vi "AutoChooseState.vi"(8 "error in (no error)":errorcluster, 9 "HotGoal?":bool, 10 "AutoMode":T2, 11 "AutoState":T1) -> (0 "error out":errorcluster, 3 "AutoState":T1)   [LabVIEW 2013]
uses:
  AutoStates.ctl
  AutoMode.ctl
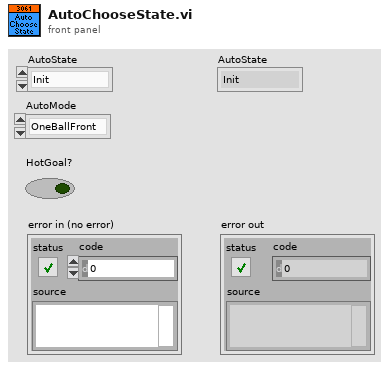
[diagram p1: front panel]
types:
  T1 = typedef "AutoStates.ctl" = enum16{"Init", "LowerArmCheckGoal", "DriveBack", "Collect", "StopCollect", "LiftArm", "RaiseServo", "Drive", "ShouldWait", "Wait", "ShootCollectorUp", "RaiseArm", "ShootCollectorDown", "Rotate1", "Rotate2", "Stop"}
  T2 = typedef "AutoMode.ctl" = enum16{"OneBallFront", "OneBallCollector", "TwoBallNormal", "TwoBallHot"}
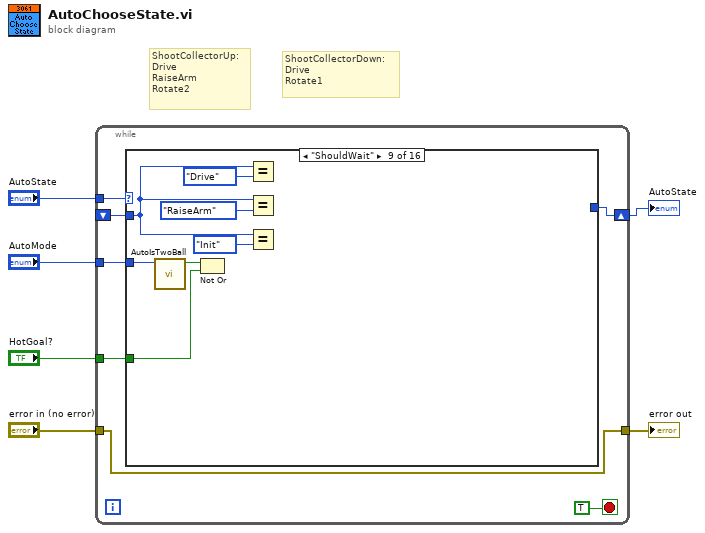
[diagram p0: block diagram]
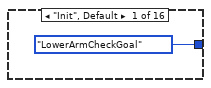
[diagram p2: hidden frame]
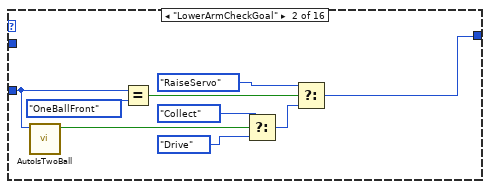
[diagram p3: hidden frame]
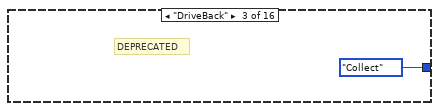
[diagram p4: hidden frame]
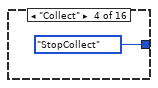
[diagram p5: hidden frame]
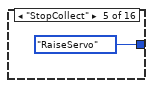
[diagram p6: hidden frame]
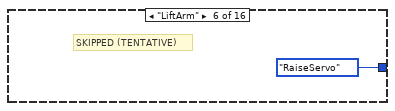
[diagram p7: hidden frame]
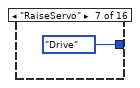
[diagram p8: hidden frame]
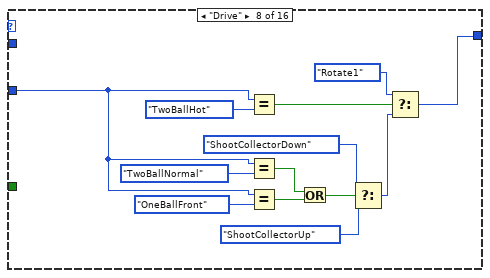
[diagram p9: hidden frame]
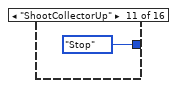
[diagram p11: hidden frame]
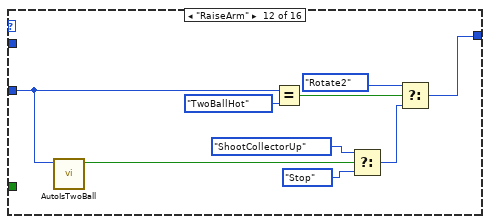
[diagram p12: hidden frame]
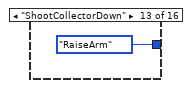
[diagram p13: hidden frame]
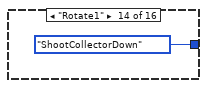
[diagram p14: hidden frame]
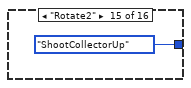
[diagram p15: hidden frame]
diagram:
  # "ShootCollectorDown:\nDrive\nRotate1"
  # "ShootCollectorUp:\nDrive\nRaiseArm\nRotate2"
  n1 = while {
    tunnel: "AutoMode" -> [w13]
    tunnel: "AutoState" -> [w12]
    tunnel: "HotGoal?" -> [w11]
    tunnel: "error in (no error)" -> [w8]
    tunnel: [w8] -> w1
    shift-right: [w10] -> w3
    shift-left: _ -> [w7]
    stop <- TRUE stop-if-true
    n2 = case shown="\"ShouldWait\"" w12 {
      selector: w12 -> [_ _ _ _ _ _ _ _ _ _ _ _ _ _ _ w62]
      tunnel: w13 -> [_ w17 _ _ _ _ _ w29 w48 _ _ w50 _ _ _ _]
      tunnel: w11 -> [_ _ _ _ _ _ _ _ w46 _ _ _ _ _ _ _]
      tunnel: [AutoStates."LowerArmCheckGoal" ("AutoState") w15 AutoStates."Collect" ("Enum") AutoStates."StopCollect" ("Enum") AutoStates."RaiseServo" ("Enum") AutoStates."RaiseServo" ("Enum") AutoStates."Drive" ("Enum") w31 _ _ AutoStates."Stop" ("f") w54 AutoStates."RaiseArm" ("Enum") AutoStates."ShootCollectorDown" ("Enum") AutoStates."ShootCollectorUp" ("Enum") w62] -> w10
      tunnel: w7 -> [_ _ _ _ _ _ _ _ w45 _ _ _ _ _ _ _]
      frame "Init", Default {
      }
      frame "LowerArmCheckGoal" {
        n3 = call "AutoIsTwoBall.vi"("AutoMode"=w17) -> ("IsTwoBall?"=w16:bool)  [unwired: 10 in]
        n4 = Equal?(x=w17, y=AutoMode."OneBallFront") -> (x = y?=w18:bool)
        n5 = Select(t=AutoStates."Collect" ("Enum"), s=w16, f=AutoStates."Drive" ("Enum")) -> (s? t:f=w20:T1)
        n6 = Select(t=AutoStates."RaiseServo" ("Enum"), s=w18, f=w20) -> (s? t:f=w15:T1)
      }
      frame "DriveBack" {
        # "DEPRECATED"
      }
      frame "Collect" {
      }
      frame "StopCollect" {
      }
      frame "LiftArm" {
        # "SKIPPED (TENTATIVE)"
      }
      frame "RaiseServo" {
      }
      frame "Drive" {
        n7 = Equal?(x=w29, y=AutoMode."TwoBallHot") -> (x = y?=w33:bool)
        n8 = Equal?(x=w29, y=AutoMode."TwoBallNormal") -> (x = y?=w40:bool)
        n9 = Equal?(x=w29, y=AutoMode."OneBallFront") -> (x = y?=w39:bool)
        n10 = Or(x=w40, y=w39) -> (x .or. y?=w35:bool)
        n11 = Select(t=AutoStates."ShootCollectorDown" ("Enum"), s=w35, f=AutoStates."ShootCollectorUp") -> (s? t:f=w34:T1)
        n12 = Select(t=AutoStates."Rotate1" ("Enum"), s=w33, f=w34) -> (s? t:f=w31:T1)
      }
      frame "ShouldWait" {
        n13 = call "AutoIsTwoBall.vi"("AutoMode"=w48) -> ("IsTwoBall?"=w47:bool)  [unwired: 10 in]
        n14 = Not Or(1:w46, 2:w47) -> ()  [unwired: 1 out]
        n15 = Equal?(x=w45, y=AutoStates."Drive") -> ()  [unwired: 1 out]
        n16 = Equal?(x=w45, y=AutoStates."RaiseArm") -> ()  [unwired: 1 out]
        n17 = Equal?(x=w45, y=AutoStates."Init") -> ()  [unwired: 1 out]
      }
      frame "Wait" {
      }
      frame "ShootCollectorUp" {
      }
      frame "RaiseArm" {
        n18 = call "AutoIsTwoBall.vi"("AutoMode"=w50) -> ("IsTwoBall?"=w53:bool)  [unwired: 10 in]
        n19 = Equal?(x=w50, y=AutoMode."TwoBallHot") -> (x = y?=w57:bool)
        n20 = Select(t=AutoStates."ShootCollectorUp" ("Enum"), s=w53, f=AutoStates."Stop" ("Enum")) -> (s? t:f=w55:T1)
        n21 = Select(t=AutoStates."Rotate2" ("Enum"), s=w57, f=w55) -> (s? t:f=w54:T1)
      }
      frame "ShootCollectorDown" {
      }
      frame "Rotate1" {
      }
      frame "Rotate2" {
      }
      frame "Stop" {
      }
    }
  }
  "AutoState" <- w3
  "error out" <- w1
